vi "CSMOMgr-Update CSMO.vi"(8 "error in (no error)":errorcluster, 10 "CSMO":T1={"info"={"Module Name"="", "Requested Name"="", "Group Name"="", "Mode"=enum."Stand Alone", "Allowed Messages"=[]}, "Refs"={"WatchDogQ"=refnum, "CSMDataDVR"=refnum, "Queue"={"HPriorityQ"=refnum, "LowPriorityQ"=refnum}, "GroupDataDVR"=refnum, "TagMap"=refnum, "ExitEvent"=refnum, "NewStateEvent"=refnum, "StatusChangeEvent"=refnum}}, 11 "CSMOMgr In":T6) -> (0 "error out":errorcluster, 2 "CSMO (Dup)":T1={"info"={"Module Name"="", "Requested Name"="", "Group Name"="", "Mode"=enum."Stand Alone", "Allowed Messages"=[]}, "Refs"={"WatchDogQ"=refnum, "CSMDataDVR"=refnum, "Queue"={"HPriorityQ"=refnum, "LowPriorityQ"=refnum}, "GroupDataDVR"=refnum, "TagMap"=refnum, "ExitEvent"=refnum, "NewStateEvent"=refnum, "StatusChangeEvent"=refnum}}, 3 "CSMOMgr Out":T6)   [LabVIEW 2017, in "Communicable State Machine.lvlib"]
uses:
  Communicable State Machine.lvlib
  CSMQ/_CSMObj.ctl
  CSMQ/_CSMObj-Info.ctl
  Typedef/_CSM_MODE.ctl
  CSMQ/_CSMObj-Refs.ctl
  CSMQ/_CSMObj-Data.ctl
  Priority Queue/Priority Queue.ctl
  Typedef/_Cross CSM State Data.ctl
  Typedef/_CSM_MSG_TYPE.ctl
  Typedef/_Cross CSM State Response.ctl
  Typedef/_CSM_Response Source Message.ctl
  Priority Queue/def-Data(LowPRI-Q).ctl
  CSMQ/_CSMObj-ModeData.ctl
  Typedef/_CSM Status Change Event Data.ctl
  Def-CSMOMgr.ctl
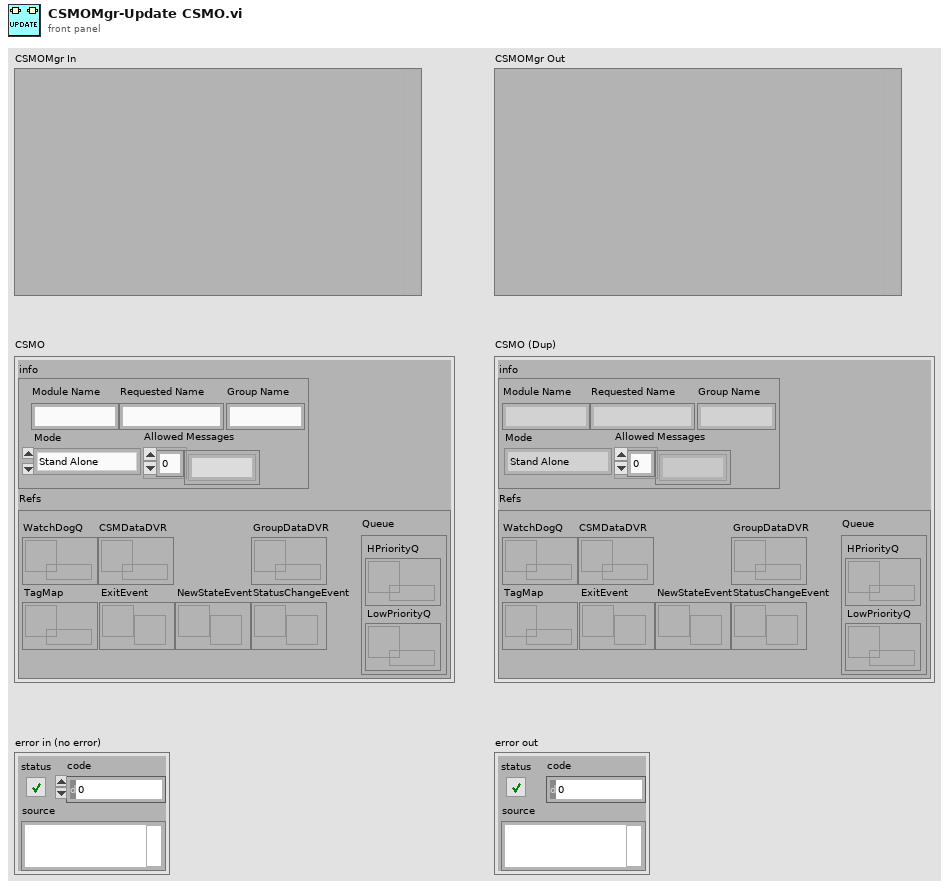
[diagram p1: front panel]
types:
  T1 = typedef "Communicable State Machine.lvlib/_CSMObj.ctl" = cluster{"info":T2, "Refs":T4}
  T2 = typedef "Communicable State Machine.lvlib/_CSMObj-Info.ctl" = cluster{"Module Name":string, "Requested Name":string, "Group Name":string, "Mode":T3, "Allowed Messages":string[]}
  T3 = typedef "Communicable State Machine.lvlib/_CSM_MODE.ctl" = enum16{"Not Exist", "Stand Alone", "CSM", "Worker", "Worker Agent", "Chain Node", "Chain"}
  T4 = typedef "Communicable State Machine.lvlib/_CSMObj-Refs.ctl" = cluster{"WatchDogQ":refnum<queue>, "CSMDataDVR":refnum<data-value>, "Queue":T5, "GroupDataDVR":refnum<data-value>, "TagMap":refnum<data-value>, "ExitEvent":refnum<user-event>, "NewStateEvent":refnum<user-event>, "StatusChangeEvent":refnum<user-event>}
  T5 = typedef "Communicable State Machine.lvlib/Priority Queue.ctl" = cluster{"HPriorityQ":refnum<queue>, "LowPriorityQ":refnum<queue>}
  T6 = typedef "Communicable State Machine.lvlib/Def-CSMOMgr.ctl" = variant
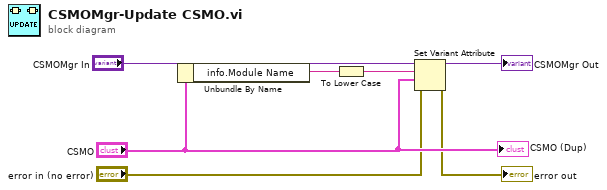
[diagram p0: block diagram]
diagram:
  n1 = Unbundle By Name("CSMO") -> ("info.Module Name"=w6:string)
  n2 = To Lower Case(string=w6) -> (all lower case string=w1:string)
  n3 = Set Variant Attribute(Variant="CSMOMgr In", name=w1, value="CSMO", error in="error in (no error)") -> (Variant out=→"CSMOMgr Out":T6, error out=→"error out":errorcluster)  [unwired: 1 out]
  "CSMO (Dup)" <- "CSMO"
